vi "Construct.vi"   [LabVIEW 2019, in "TSC Event Logger.lvlib" / "Text File - Binary.lvclass"]
doc: "Polymorphic, selectable constructor for a Binary text file sink.\n\n<b>Code Developed By:</b>\nTechnology Service Corporation\nBloomington, IN 47403\nwww.tsc.com/atcs\n\nDeveloper:\nDaniel Coons"
uses:
  Text File - Binary.lvclass
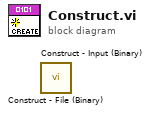
[diagram p0: block diagram]
diagram:
  n1 = call "Construct - Input (Binary).vi"() -> ()  [unwired: 10 in, 2 out]
  n2 = call "Construct - File (Binary).vi"() -> ()  [unwired: 10 in, 2 out]
